vi "Updated Dynamic Headers.vi"(8 "Old Data":string[](array[string])=["Full Path", "Batch Path", "Folder Name"], 9 "New Data":string[](array[string])=["Full Path", "Batch Path", "Folder Name"], 10 "This Data's Headers":string[](array[string])=["Full Path", "Batch Path", "Folder Name"], 11 "Old Headers":string[](array[string])=["Full Path", "Batch Path", "Folder Name"]) -> (1 "Formatted New Data":string[](array[string])=["Full Path", "Batch Path", "Folder Name"], 3 "Merged Headers":string[](array[string]))   [LabVIEW 2010]
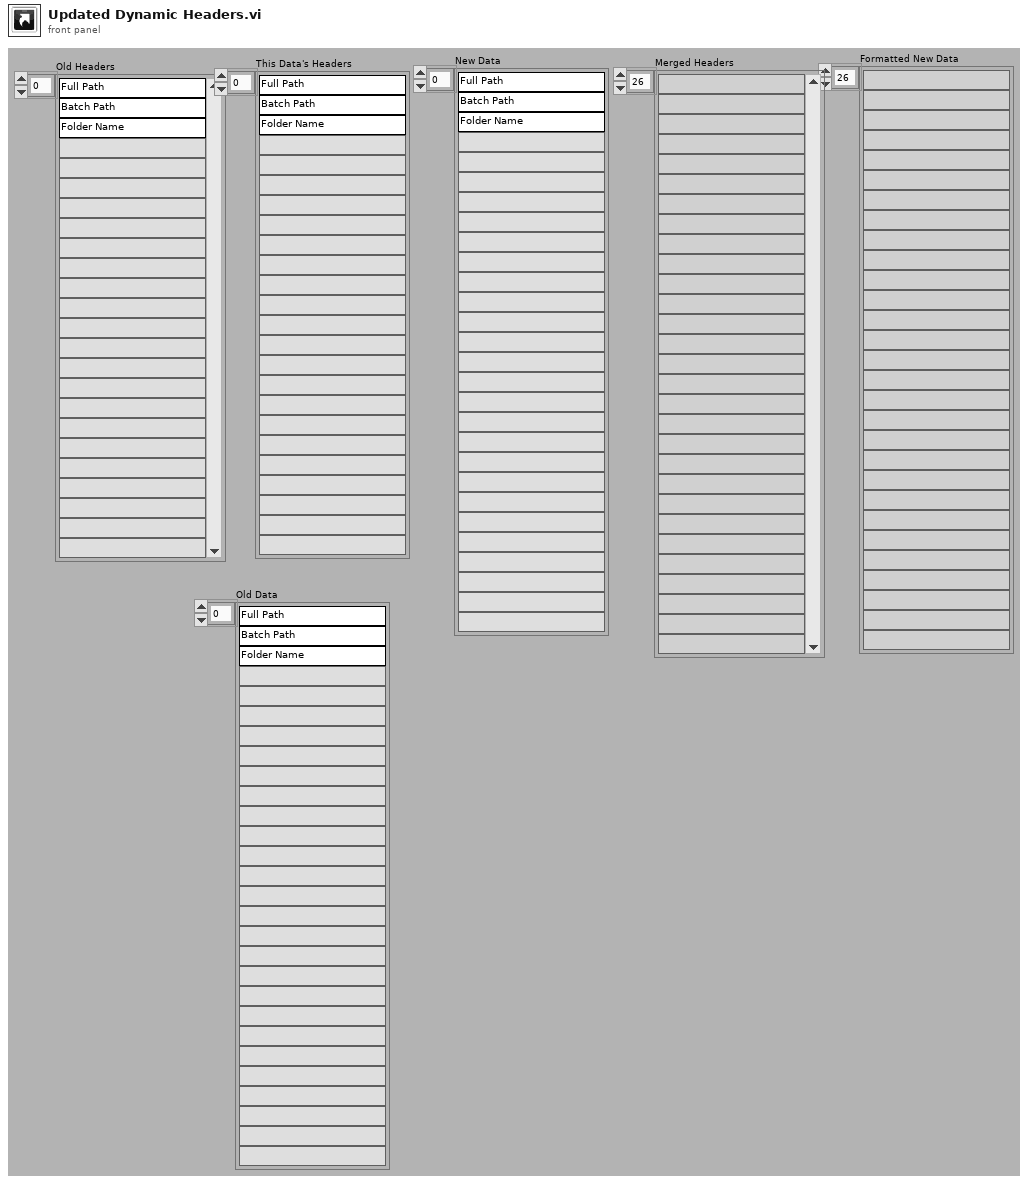
[diagram p1: front panel]
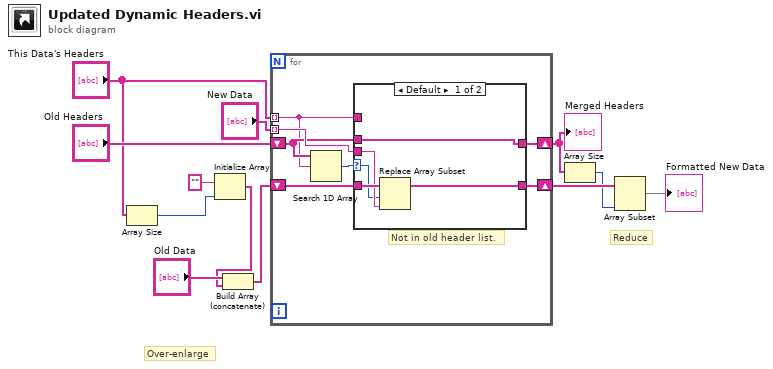
[diagram p0: block diagram]
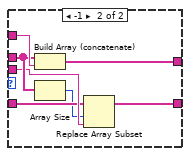
[diagram p2: hidden frame]
diagram:
  # "Reduce"
  # "Over-enlarge"
  n1 = Array Size(array="This Data's Headers") -> (size(s)=w1:i32)
  n2 = Initialize Array("", w1) -> (w2:string[])
  n3 = Build Array (concatenate)("Old Data", w2) -> (w3:string[])
  n4 = for {
    tunnel: "This Data's Headers" -> [w14] mode=indexing
    tunnel: "New Data" -> [w18] mode=indexing
    shift-right: [w17] -> w8
    shift-left: w3 -> [w19]
    shift-right: [w16] -> w7
    shift-left: "Old Headers" -> [w15]
    # "Not in old header list."
    n5 = Search 1D Array(1D array=w15, element=w14) -> (index of element=w13:i32)  [unwired: 1 in]
    n6 = case shown="Default" w13 {
      selector: w13 -> [w22 _]
      tunnel: w19 -> [w24 w27]
      tunnel: w18 -> [w23 w28]
      tunnel: [w21 w26] -> w17
      tunnel: [w20 w30] -> w16
      tunnel: w15 -> [w20 w29]
      tunnel: w14 -> [_ w31]
      frame Default {
        n7 = Replace Array Subset(array=w24, new element=w23, index=w22) -> (w21:string[])
      }
      frame -1 {
        n8 = Build Array (concatenate)(w29, w31) -> (w30:string[])
        n9 = Array Size(array=w29) -> (size(s)=w25:i32)
        n10 = Replace Array Subset(array=w27, new element=w28, index=w25) -> (w26:string[])
      }
    }
  }
  "Merged Headers" <- w7
  n11 = Array Size(array=w7) -> (size(s)=w6:i32)
  n12 = Array Subset(array=w8, length=w6) -> (→"Formatted New Data":string[])  [unwired: 1 in]
